vi "AlGaAs_GaAs_SL_v01.vi"(2 "Debug Mode":bool, 3 "Elapsed Time(s)":dbl, 4 "State":enum16{"Edit", "Start", "Run", "End", "Idle"}(ring), 5 "Argument List In":string[](array[string])) -> (0 "Status Out":string, 1 "Argument List Out":string[](array[string]))   [LabVIEW 2011]
panel:
  in  "fGa dilution":dbl
  in  "Tab Control":enum32{"Step 1", "Step 2"}(tab)
  in  "Al flow (0-100 sccm)":dbl format="%.1f"
  in  "tFlow (s)":dbl
  in  "tWait (s)":dbl
  in  "Ga flow (0-10 sccm)":dbl format="%.3f"
  in  "Ga flow (0-10 sccm)":dbl format="%.3f"
  in  "tFlow (s)":dbl
  in  "tWait (s)":dbl
  out "tphase(s)":dbl[](array[numeric])
  out "nstep":dbl
  out "phase":i32
  out "done":bool
  in  "nPeriods":dbl
  out "tTotal(s)":dbl
  out "tPeriod(s)":dbl
  in  "Cancel":bool
  in  "OK":bool
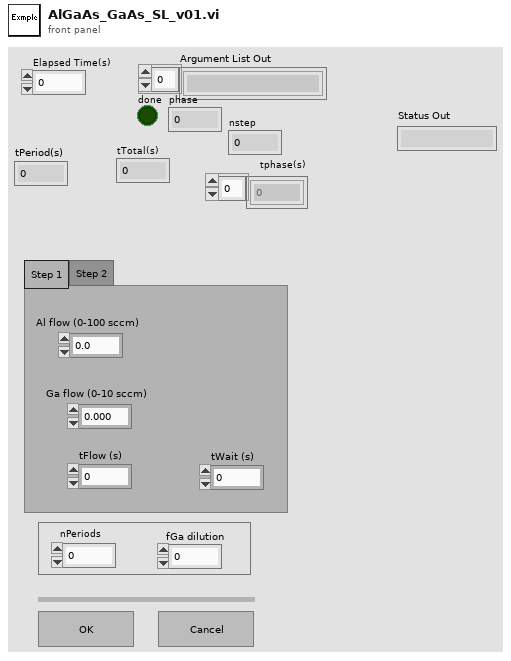
[diagram p1: front panel]
types:
  T1 = enum16{"Discrete", "Continuous", "Instantaneous"}
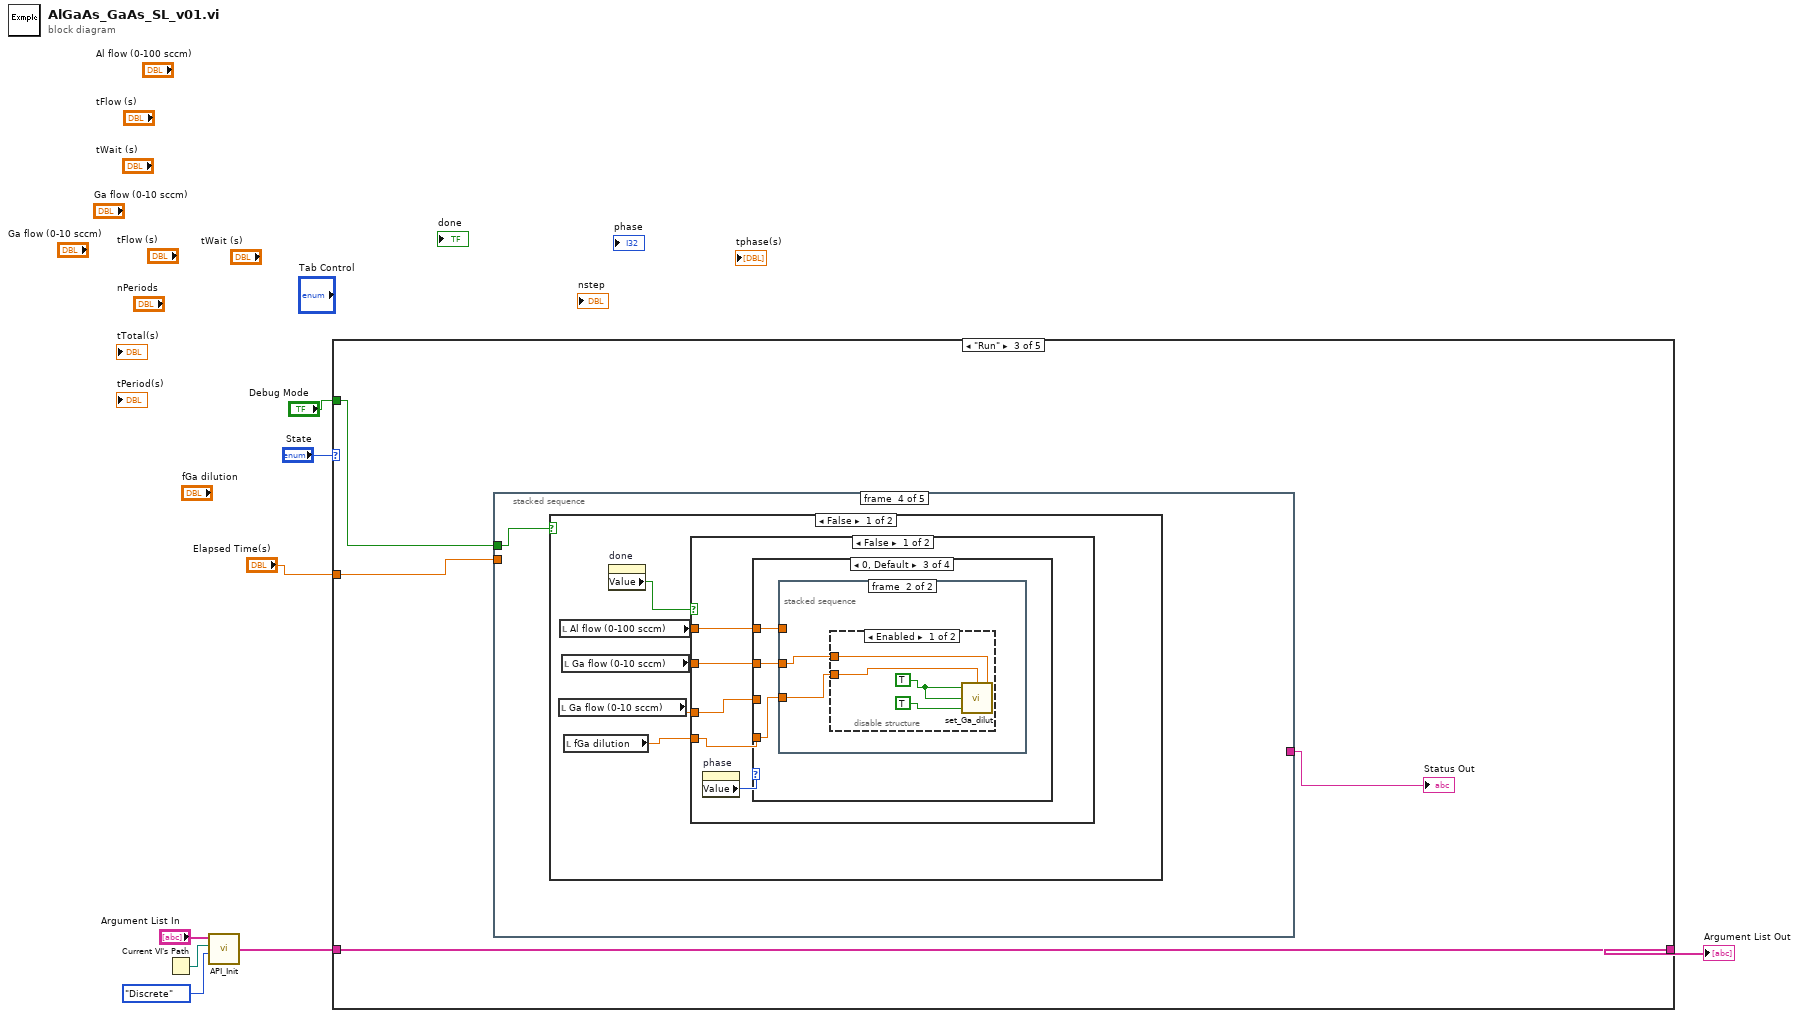
[diagram p0: block diagram]
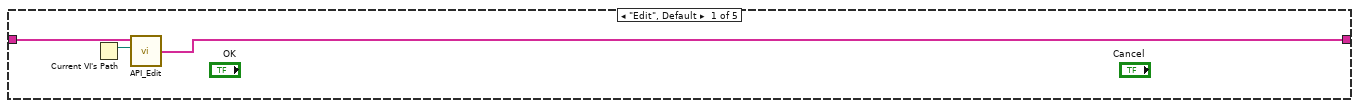
[diagram p2: hidden frame]
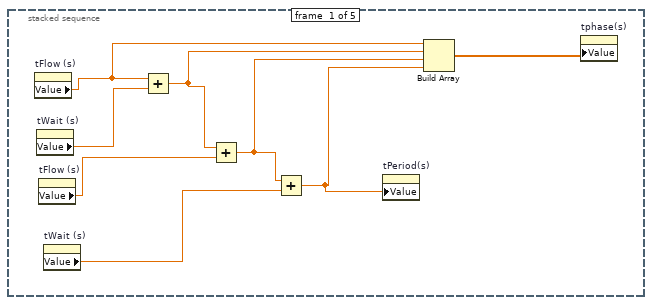
[diagram p4: hidden frame]
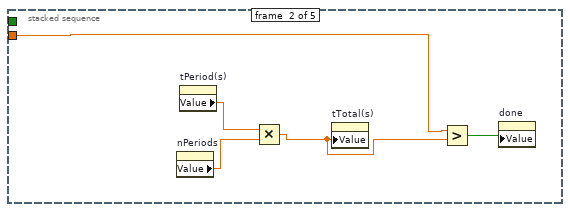
[diagram p5: hidden frame]
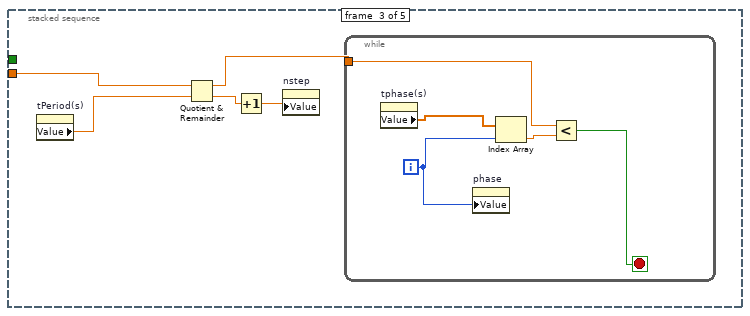
[diagram p6: hidden frame]
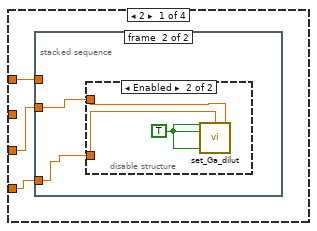
[diagram p7: hidden frame]
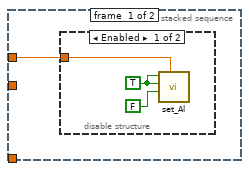
[diagram p8: hidden frame]
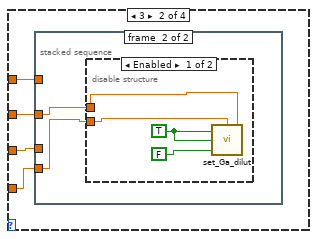
[diagram p11: hidden frame]
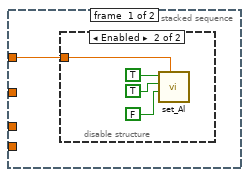
[diagram p12: hidden frame]
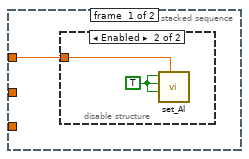
[diagram p15: hidden frame]
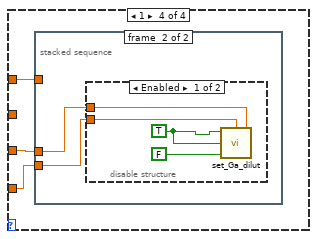
[diagram p18: hidden frame]
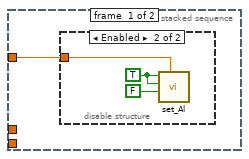
[diagram p19: hidden frame]
diagram:
  n1 = Current VI's Path() -> (path=w5:path)
  n2 = call "API_Init.vi"("API Mode"=T1."Discrete", "VI Path"=w5, "Argument List In"="Argument List In") -> ("Argument List Out"=w6:string[])  [unwired: 1 in]
  n3 = case shown="\"Run\"" "State" {
    tunnel: [w9 w12 w16 w150 w151] -> w2
    tunnel: w6 -> [w11 w12 w16 w150 w151]
    tunnel: "Debug Mode" -> [_ _ w14 _ _]
    tunnel: "Elapsed Time(s)" -> [_ _ w15 _ _]
    frame "Edit", Default {
      n4 = Current VI's Path() -> (path=w10:path)
      n5 = call "API_Edit.vi"("VI Path"=w10, "Argument List In"=w11) -> ("Argument List Out"=w9:string[])  [unwired: 2 in]
    }
    frame "Start" {
    }
    frame "Run" {
      n6 = stacked-sequence {
        tunnel: w15 -> [_ w27 w34 _ _]
        tunnel: w14 -> [_ _ _ w40 _]
        tunnel: [_ _ _ _ w113] -> w13
        frame #0 {
          n7 = property on="tFlow (s)" class="DigNum (strict)"() -> ("Value"=w23:dbl)  [unwired: 2 in, 2 out]
          n8 = property on="tWait (s)" class="DigNum (strict)"() -> ("Value"=w24:dbl)  [unwired: 2 in, 2 out]
          n9 = property on="tFlow (s)" class="DigNum (strict)"() -> ("Value"=w21:dbl)  [unwired: 2 in, 2 out]
          n10 = property on="tWait (s)" class="DigNum (strict)"() -> ("Value"=w20:dbl)  [unwired: 2 in, 2 out]
          n11 = Add(x=w23, y=w24) -> (x+y=w22:dbl)
          n12 = Add(x=w22, y=w21) -> (x+y=w19:dbl)
          n13 = Add(x=w19, y=w20) -> (x+y=w18:dbl)
          n14 = property on="tPeriod(s)" class="DigNum (strict)"("Value"=w18) -> ()  [unwired: 2 in, 2 out]
          n15 = Build Array(w23, w22, w19, w18) -> (w17:dbl[])
          n16 = property on="tphase(s)" class="Arr (strict)"("Value"=w17) -> ()  [unwired: 2 in, 2 out]
        }
        frame #1 {
          n17 = property on="nPeriods" class="DigNum (strict)"() -> ("Value"=w28:dbl)  [unwired: 2 in, 2 out]
          n18 = property on="tPeriod(s)" class="DigNum (strict)"() -> ("Value"=w29:dbl)  [unwired: 2 in, 2 out]
          n19 = Multiply(x=w29, y=w28) -> (x*y=w26:dbl)
          n20 = property on="tTotal(s)" class="DigNum (strict)"("Value"=w26) -> ()  [unwired: 2 in, 2 out]
          n21 = Greater?(x=w27, y=w26) -> (0:w25:bool)
          n22 = property on="done" class="Bool (strict)"("Value"=w25) -> ()  [unwired: 2 in, 2 out]
        }
        frame #2 {
          n23 = property on="tPeriod(s)" class="DigNum (strict)"() -> ("Value"=w33:dbl)  [unwired: 2 in, 2 out]
          n24 = Quotient & Remainder(x=w34, y=w33) -> (x-y*floor(x/y)=w32:dbl, floor(x/y)=w31:dbl)
          n25 = Increment(x=w31) -> (x+1=w30:dbl)
          n26 = property on="nstep" class="DigNum (strict)"("Value"=w30) -> ()  [unwired: 2 in, 2 out]
          n27 = while {
            tunnel: w32 -> [w38]
            i -> [w36]
            stop <- w35 stop-if-true
            n28 = property on="tphase(s)" class="Arr (strict)"() -> ("Value"=w39:dbl[])  [unwired: 2 in, 2 out]
            n29 = property on="phase" class="DigNum (strict)"("Value"=w36) -> ()  [unwired: 2 in, 2 out]
            n30 = Index Array(array=w39, index=w36) -> (element=w37:dbl)
            n31 = Less?(x=w38, y=w37) -> (x < y?=w35:bool)
          }
        }
        frame #3 {
          n32 = case shown="False" w40 {
            frame False {
              n33 = local read "Ga flow (0-10 sccm)"() -> (w45:dbl)
              n34 = local read "Al flow (0-100 sccm)"() -> (w44:dbl)
              n35 = local read "Ga flow (0-10 sccm)"() -> (w42:dbl)
              n36 = local read "fGa dilution"() -> (w41:dbl)
              n37 = property on="done" class="Bool (strict)"() -> ("Value"=w43:bool)  [unwired: 2 in, 2 out]
              n38 = case shown="False" w43 {
                tunnel: w45 -> [w50 w103]
                tunnel: w44 -> [w49 w104]
                tunnel: w42 -> [w47 _]
                tunnel: w41 -> [w46 _]
                frame False {
                  n39 = property on="phase" class="DigNum (strict)"() -> ("Value"=w48:i32)  [unwired: 2 in, 2 out]
                  n40 = case shown="0, Default" w48 {
                    tunnel: w49 -> [w53 w66 w80 w92]
                    tunnel: w50 -> [w52 w65 _ w91]
                    tunnel: w47 -> [_ w64 w79 _]
                    tunnel: w46 -> [w51 w63 w78 w90]
                    frame 2 {
                      n41 = stacked-sequence {
                        tunnel: w53 -> [w54 _]
                        tunnel: w52 -> [_ w59]
                        tunnel: w51 -> [_ w58]
                        frame #0 {
                          n42 = disable-structure shown="Enabled" {
                            disable-tunnel: w54 -> [w55 _]
                            frame Enabled {
                              w57 = TRUE ("Ga Active")
                              n43 = call "set_Al.vi"("Aluminum Flow"=w55, "Al Run"=FALSE, "Al Bubbler"=w57, "Al Active"=w57) -> ()  [unwired: 6 in]
                            }
                            frame Disabled {
                            }
                          }
                        }
                        frame #1 {
                          n44 = disable-structure shown="Enabled" {
                            disable-tunnel: w59 -> [_ w62]
                            disable-tunnel: w58 -> [_ w61]
                            frame Disabled {
                            }
                            frame Enabled {
                              w60 = TRUE ("Ga Active")
                              n45 = call "set_Ga_dilut.vi"("Ga flow (0-10 sccm)"=w62, "fDilution"=w61, "Run"=w60, "Bubbler In"=w60, "Active"=w60) -> ()
                            }
                          }
                        }
                      }
                    }
                    frame 3 {
                      n46 = stacked-sequence {
                        tunnel: w66 -> [w67 _]
                        tunnel: w65 -> [_ _]
                        tunnel: w64 -> [_ w73]
                        tunnel: w63 -> [_ w72]
                        frame #0 {
                          n47 = disable-structure shown="Enabled" {
                            disable-tunnel: w67 -> [_ w68]
                            frame Disabled {
                            }
                            frame Enabled {
                              n48 = call "set_Al.vi"("Aluminum Flow"=w68, "Al Run"=FALSE, "Al Bubbler"=TRUE, "Al Active"=TRUE) -> ()  [unwired: 6 in]
                            }
                          }
                        }
                        frame #1 {
                          n49 = disable-structure shown="Enabled" {
                            disable-tunnel: w73 -> [w77 _]
                            disable-tunnel: w72 -> [w76 _]
                            frame Enabled {
                              w75 = TRUE ("Ga Active")
                              n50 = call "set_Ga_dilut.vi"("Ga flow (0-10 sccm)"=w77, "fDilution"=w76, "Run"=FALSE ("Ga Run"), "Bubbler In"=w75, "Active"=w75) -> ()
                            }
                            frame Disabled {
                            }
                          }
                        }
                      }
                    }
                    frame 0, Default {
                      n51 = stacked-sequence {
                        tunnel: w80 -> [w81 _]
                        tunnel: w79 -> [_ w85]
                        tunnel: w78 -> [_ w84]
                        frame #0 {
                          n52 = disable-structure shown="Enabled" {
                            disable-tunnel: w81 -> [_ w83]
                            frame Disabled {
                            }
                            frame Enabled {
                              w82 = TRUE ("Al Active")
                              n53 = call "set_Al.vi"("Aluminum Flow"=w83, "Al Run"=w82, "Al Bubbler"=w82, "Al Active"=w82) -> ()  [unwired: 6 in]
                            }
                          }
                        }
                        frame #1 {
                          n54 = disable-structure shown="Enabled" {
                            disable-tunnel: w85 -> [w89 _]
                            disable-tunnel: w84 -> [w86 _]
                            frame Enabled {
                              w88 = TRUE ("Ga Active")
                              n55 = call "set_Ga_dilut.vi"("Ga flow (0-10 sccm)"=w89, "fDilution"=w86, "Run"=TRUE ("Ga Run"), "Bubbler In"=w88, "Active"=w88) -> ()
                            }
                            frame Disabled {
                            }
                          }
                        }
                      }
                    }
                    frame 1 {
                      n56 = stacked-sequence {
                        tunnel: w91 -> [_ w98]
                        tunnel: w92 -> [w93 _]
                        tunnel: w90 -> [_ w97]
                        frame #0 {
                          n57 = disable-structure shown="Enabled" {
                            disable-tunnel: w93 -> [_ w95]
                            frame Disabled {
                            }
                            frame Enabled {
                              w94 = TRUE ("Al Bubbler")
                              n58 = call "set_Al.vi"("Aluminum Flow"=w95, "Al Run"=FALSE, "Al Bubbler"=w94, "Al Active"=w94) -> ()  [unwired: 6 in]
                            }
                          }
                        }
                        frame #1 {
                          n59 = disable-structure shown="Enabled" {
                            disable-tunnel: w98 -> [w100 _]
                            disable-tunnel: w97 -> [w99 _]
                            frame Enabled {
                              w101 = TRUE ("Ga Active")
                              n60 = call "set_Ga_dilut.vi"("Ga flow (0-10 sccm)"=w100, "fDilution"=w99, "Run"=FALSE ("Ga Run"), "Bubbler In"=w101, "Active"=w101) -> ()
                            }
                            frame Disabled {
                            }
                          }
                        }
                      }
                    }
                  }
                }
                frame True {
                  n61 = stacked-sequence {
                    tunnel: w104 -> [w105 _]
                    tunnel: w103 -> [_ w109]
                    frame #0 {
                      n62 = disable-structure shown="Enabled" {
                        disable-tunnel: w105 -> [_ w108]
                        frame Disabled {
                        }
                        frame Enabled {
                          w107 = TRUE ("Al Active")
                          n63 = call "set_Al.vi"("Aluminum Flow"=w108, "Al Run"=FALSE, "Al Bubbler"=w107, "Al Active"=w107) -> ()  [unwired: 6 in]
                        }
                      }
                    }
                    frame #1 {
                      n64 = disable-structure shown="Enabled" {
                        disable-tunnel: w109 -> [w110 _]
                        frame Enabled {
                          w111 = TRUE ("Ga Active")
                          n65 = call "set_Ga.vi"("Ga Active"=w111, "Ga Flow 1"=w110, "Ga Bubbler"=w111, "Ga Run"=FALSE) -> ()  [unwired: 4 in, 8 out]
                        }
                        frame Disabled {
                        }
                      }
                    }
                  }
                }
              }
            }
            frame True {
            }
          }
        }
        frame #4 {
          n66 = property on="done" class="Bool (strict)"() -> ("Value"=w114:bool)  [unwired: 2 in, 2 out]
          n67 = case shown="False" w114 {
            tunnel: [w115 w149] -> w113
            frame False {
              n68 = property on="phase" class="DigNum (strict)"() -> ("Value"=w122:i32)  [unwired: 2 in, 2 out]
              n69 = case shown="0, Default" w122 {
                tunnel: [w125 "wait (GaAs)" w131 "wait (AlGaAs)"] -> w121
                frame 2 {
                  n70 = local read "Ga flow (0-10 sccm)"() -> (w124:dbl)
                  n71 = Format Into String(format string="%4.2f", w124) -> (resulting string=w128:string)  [unwired: 2 in, 1 out]
                  n72 = Concatenate Strings("Ga(" ("string"), w128, "sccm)" ("string")) -> (w125:string)
                }
                frame 3 {
                }
                frame 0, Default {
                  n73 = local read "Al flow (0-100 sccm)"() -> (w138:dbl)
                  n74 = local read "Ga flow (0-10 sccm)"() -> (w137:dbl)
                  n75 = Format Into String(format string="%4.1f", w138) -> (resulting string=w140:string)  [unwired: 2 in, 1 out]
                  n76 = Format Into String(format string="%4.1f", w137) -> (resulting string=w133:string)  [unwired: 2 in, 1 out]
                  n77 = Concatenate Strings("Al(" ("string"), w140, "sccm)" ("string")) -> (w132:string)
                  n78 = Concatenate Strings(w132, "Ga(" ("string"), w133, "sccm)" ("string")) -> (w131:string)
                }
                frame 1 {
                }
              }
              n79 = property on="nstep" class="DigNum (strict)"() -> ("Value"=w123:dbl)  [unwired: 2 in, 2 out]
              n80 = Format Into String(format string="%3.0f", w123) -> (resulting string=w118:string)  [unwired: 2 in, 1 out]
              n81 = Concatenate Strings("Period " ("string"), w118) -> (w116:string)
              n82 = Concatenate Strings(w116, ", " ("string"), w121) -> (w115:string)
            }
            frame True {
              n83 = property on="nPeriods" class="DigNum (strict)"() -> ("Value"=w144:dbl)  [unwired: 2 in, 2 out]
              n84 = Format Into String(format string="%3.0f", w144) -> (resulting string=w145:string)  [unwired: 2 in, 1 out]
              n85 = Concatenate Strings("done after", w145, " periods" ("string")) -> (w149:string)
            }
          }
        }
      }
      "Status Out" <- w13
    }
    frame "End" {
    }
    frame "Idle" {
    }
  }
  "Argument List Out" <- w2
